vi "Win_RS232_Config.vi"(8 "error in":errorcluster caption="错误输入") -> (0 "error out":errorcluster caption="错误输出", 1 "Yes out":bool=TRUE)   [LabVIEW 2020]
uses:
  <vilib>/Utility/xml.llb/Write to XML File(array).vi
panel:
  out "CommNameOut":T1={"ACCCommName"="COM6", "HostCommName"="COM4"}
  out "Serial Configuration Out":T2={"ACC Serial Configuration"={"Baud Rate"=9600, "Parity"=0, "Data Bits"=8, "Stop Bits"=10, "Flow Control"=0}, "Host ACC Serial Configuration"={"Baud Rate"=9600, "Parity"=0, "Data Bits"=8, "Stop Bits"=10, "Flow Control"=0}} {"Host ACC Serial Configuration"."Flow Control" items=["None", "XON/XOFF", "RTS/CTS", "XON/XOFF & RTS/CTS", "DTR/DSR", "XON/XOFF & DTR/DSR"]; "Host ACC Serial Configuration"."Stop Bits" items=["1.0"=10, "1.5"=15, "2.0"=20]; "Host ACC Serial Configuration"."Data Bits" items=["7"=7, "8"=8]; "Host ACC Serial Configuration"."Parity" items=["None", "Odd", "Even", "Mark", "Space"]; "Host ACC Serial Configuration"."Baud Rate" items=["300"=300, "600"=600, "1200"=1200, "2400"=2400, "4800"=4800, "9600"=9600, "19200"=19200]; "ACC Serial Configuration"."Flow Control" items=["None", "XON/XOFF", "RTS/CTS", "XON/XOFF & RTS/CTS", "DTR/DSR", "XON/XOFF & DTR/DSR"]; "ACC Serial Configuration"."Stop Bits" items=["1.0"=10, "1.5"=15, "2.0"=20]; "ACC Serial Configuration"."Data Bits" items=["7"=7, "8"=8]; "ACC Serial Configuration"."Parity" items=["None", "Odd", "Even", "Mark", "Space"]; "ACC Serial Configuration"."Baud Rate" items=["300"=300, "600"=600, "1200"=1200, "2400"=2400, "4800"=4800, "9600"=9600, "19200"=19200]}
  in  "HostStopBits:":u16(ring)=10 caption="StopBits:" items=["1.0"=10, "1.5"=15, "2.0"=20]
  in  "HostDataBits:":u16(ring)=8 caption="DataBits:" items=["5"=5, "6"=6, "7"=7, "8"=8]
  in  "HostParity:":u16(ring) caption="Parity:" items=["None", "Odd", "Even", "Mark", "Space"]
  in  "HostBaudRate:":u16(ring)=9600 caption="BaudRate:" items=["1200"=1200, "2400"=2400, "4800"=4800, "9600"=9600, "14400"=14400, "19200"=19200, "28800"=28800, "38400"=38400, "57600"=57600, "115200"=0]
  in  "HostCommName:":refnum<visa-resource-name>="COM4" caption="CommName:"
  in  "No":bool
  in  "Yes":bool
  in  "ACCStopBits:":u16(ring)=10 caption="StopBits:" items=["1.0"=10, "1.5"=15, "2.0"=20]
  in  "ACCDataBits:":u16(ring)=8 caption="DataBits:" items=["5"=5, "6"=6, "7"=7, "8"=8]
  in  "ACCParity:":u16(ring) caption="Parity:" items=["None", "Odd", "Even", "Mark", "Space"]
  in  "ACCBaudRate:":u16(ring)=9600 caption="BaudRate:" items=["1200"=1200, "2400"=2400, "4800"=4800, "9600"=9600, "14400"=14400, "19200"=19200, "28800"=28800, "38400"=38400, "57600"=57600, "115200"=0]
  in  "ACCCommName:":refnum<visa-resource-name>="COM6" caption="CommName:"
  # "ACC"
  # "Host"
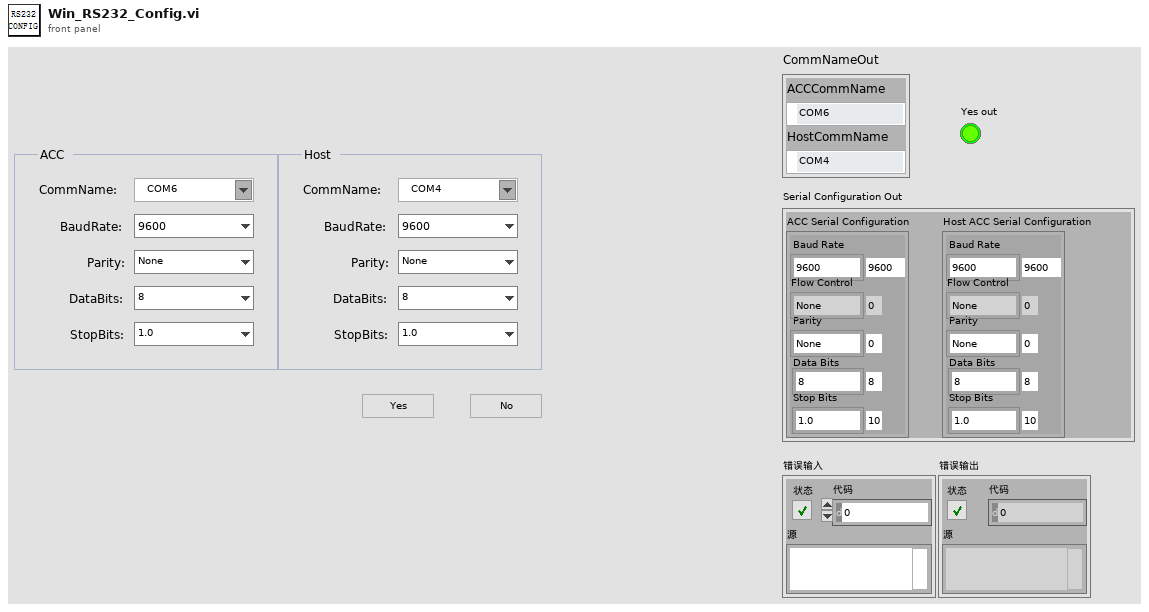
[diagram p1: front panel]
types:
  T1 = cluster{"ACCCommName":refnum<visa-resource-name>, "HostCommName":refnum<visa-resource-name>}
  T2 = cluster{"ACC Serial Configuration":cluster{"Baud Rate":u32, "Parity":u16, "Data Bits":u16, "Stop Bits":u16, "Flow Control":u16}, "Host ACC Serial Configuration":cluster{"Baud Rate":u32, "Parity":u16, "Data Bits":u16, "Stop Bits":u16, "Flow Control":u16}}
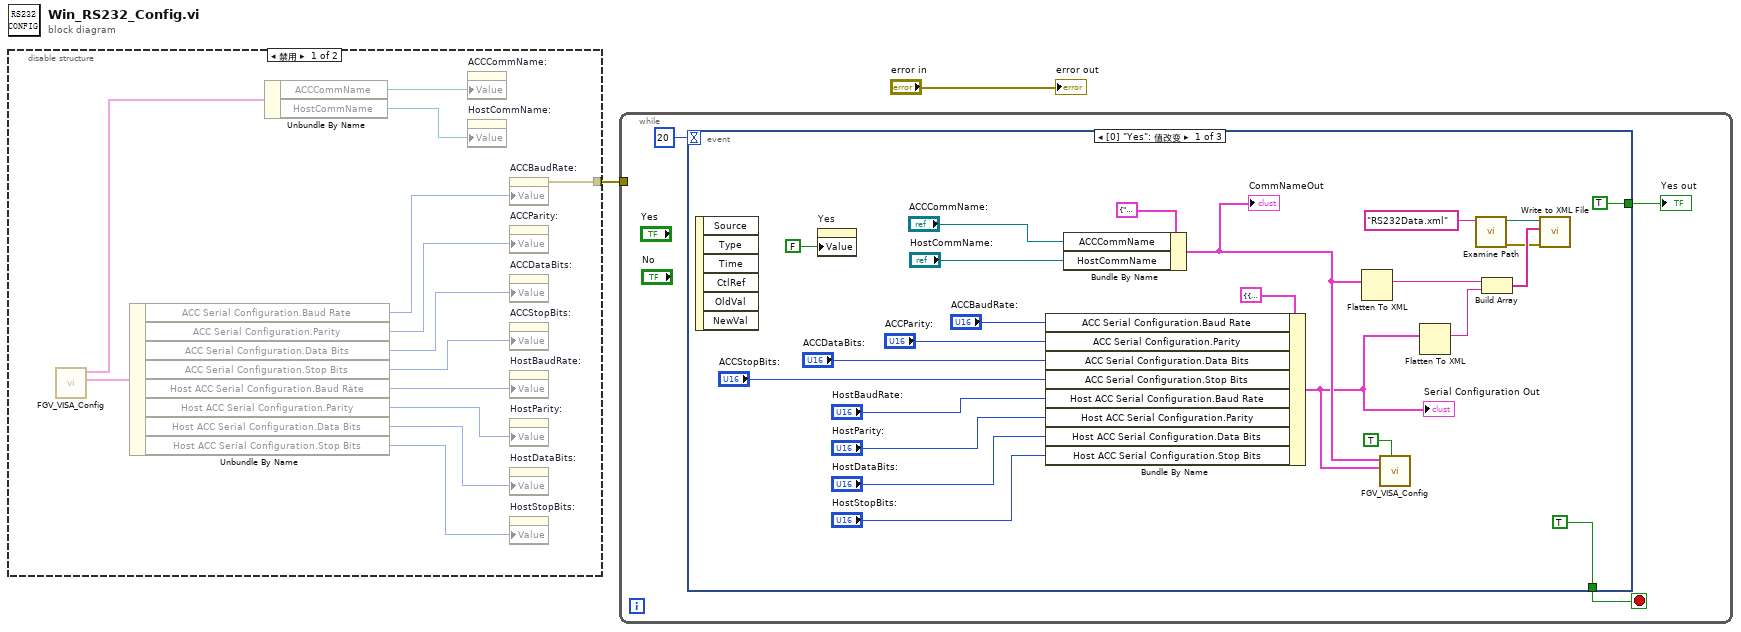
[diagram p0: block diagram]
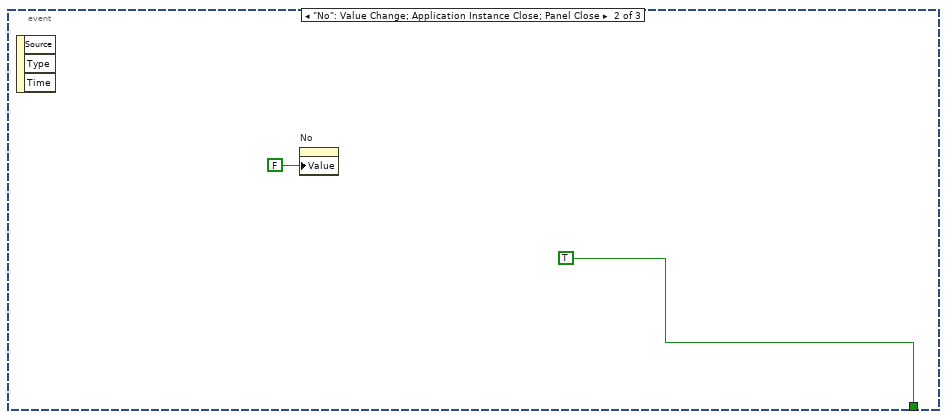
[diagram p3: hidden frame]
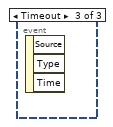
[diagram p4: hidden frame]
diagram:
  n1 = disable-structure shown="禁用" {
    disable-tunnel: [w15 _] -> w1
    frame Disabled {
      n2 = call "FGV_VISA_Config.vi"() -> ("Serial Configuration Out"=w11:T2, "CommNameOut"=w14:T1)  [unwired: 9 in, 1 out]
      n3 = Unbundle By Name(w11) -> ("ACC Serial Configuration.Baud Rate"=w10:u32, "ACC Serial Configuration.Parity"=w9:u16, "ACC Serial Configuration.Data Bits"=w8:u16, "ACC Serial Configuration.Stop Bits"=w7:u16, "Host ACC Serial Configuration.Baud Rate"=w6:u32, "Host ACC Serial Configuration.Parity"=w5:u16, "Host ACC Serial Configuration.Data Bits"=w4:u16, "Host ACC Serial Configuration.Stop Bits"=w3:u16)
      n4 = Unbundle By Name(w14) -> ("ACCCommName"=w13:refnum<visa-resource-name>, "HostCommName"=w12:refnum<visa-resource-name>)
      n5 = property on="ACCCommName:" class="VISAName"("Value"=w13) -> ()  [unwired: 2 in, 2 out]
      n6 = property on="HostCommName:" class="VISAName"("Value"=w12) -> ()  [unwired: 2 in, 2 out]
      n7 = property on="ACCBaudRate:" class="Ring (严格)"("Value"=w10) -> (error out=w15:errorcluster)  [unwired: 2 in, 1 out]
      n8 = property on="ACCParity:" class="Ring (严格)"("Value"=w9) -> ()  [unwired: 2 in, 2 out]
      n9 = property on="ACCDataBits:" class="Ring (严格)"("Value"=w8) -> ()  [unwired: 2 in, 2 out]
      n10 = property on="ACCStopBits:" class="Ring (严格)"("Value"=w7) -> ()  [unwired: 2 in, 2 out]
      n11 = property on="HostBaudRate:" class="Ring (严格)"("Value"=w6) -> ()  [unwired: 2 in, 2 out]
      n12 = property on="HostParity:" class="Ring (严格)"("Value"=w5) -> ()  [unwired: 2 in, 2 out]
      n13 = property on="HostDataBits:" class="Ring (严格)"("Value"=w4) -> ()  [unwired: 2 in, 2 out]
      n14 = property on="HostStopBits:" class="Ring (严格)"("Value"=w3) -> ()  [unwired: 2 in, 2 out]
    }
    frame Enabled {
    }
  }
  n15 = while {
    tunnel: w1 -> [_]
    stop <- w17 stop-if-true
    n16 = event shown="[0] \"Yes\": 值改变" {
      selector: _ -> [_ _ _]
      dyn-events: _ -> [_ _ _]
      timeout: 20 -> [_ _ _]
      tunnel: [TRUE TRUE _] -> w17
      tunnel: [TRUE _ _] -> w16
      event "Yes": Value Change {
        n17 = event-data() -> ()  [unwired: 1 in, 6 out]
        n18 = property on="Yes" class="Bool (严格)"("Value"=FALSE ("Yes")) -> ()  [unwired: 2 in, 2 out]
        n19 = Bundle By Name(cluster=T2 {"ACC Serial Configuration"={"Baud Rate"=9600, "Parity"=0, "Data Bits"=8, "Stop Bits"=10, "Flow Control"=0}, "Host ACC Serial Configuration"={"Baud Rate"=9600, "Parity"=0, "Data Bits"=8, "Stop Bits"=10, "Flow Control"=0}} ("Serial Configuration Out"), "ACC Serial Configuration.Baud Rate"="ACCBaudRate:", "ACC Serial Configuration.Parity"="ACCParity:", "ACC Serial Configuration.Data Bits"="ACCDataBits:", "ACC Serial Configuration.Stop Bits"="ACCStopBits:", "Host ACC Serial Configuration.Baud Rate"="HostBaudRate:", "Host ACC Serial Configuration.Parity"="HostParity:", "Host ACC Serial Configuration.Data Bits"="HostDataBits:", "Host ACC Serial Configuration.Stop Bits"="HostStopBits:") -> (w19:T2)
        "Serial Configuration Out" <- w19
        n20 = Bundle By Name(cluster=T1 {"ACCCommName"="COM4", "HostCommName"="COM4"} ("CommNameOut"), "ACCCommName"="ACCCommName:", "HostCommName"="HostCommName:") -> (w20:T1)
        "CommNameOut" <- w20
        n21 = Flatten To XML(6:w20) -> (2:w34:string)
        n22 = call "FGV_VISA_Config.vi"("Write?"=TRUE, "Serial Configuration"=w19, "CommName"=w20) -> ()  [unwired: 6 in, 3 out]
        n23 = Flatten To XML(6:w19) -> (2:w33:string)
        n24 = call "Examine Path.vi"("Filename"="RS232Data.xml") -> ("error out"=w30:errorcluster, "Path"=w32:path)  [unwired: 9 in]
        n25 = Build Array(w34, w33) -> (w31:string[])
        n26 = call-poly <vilib>:"Write to XML File.vi"("error in (no error)"=w30, "XML Input"=w31, "XML File Path"=w32) -> ()  [unwired: 6 in, 3 out]
      }
      event "No": Value Change; Application Instance Close; Panel Close {
        n27 = event-data() -> ()  [unwired: 1 in, 3 out]
        n28 = property on="No" class="Bool (严格)"("Value"=FALSE ("No")) -> ()  [unwired: 2 in, 2 out]
      }
      event Timeout {
        n29 = event-data() -> ()  [unwired: 1 in, 3 out]
      }
    }
    "Yes out" <- w16
  }
  "error out" <- "error in"
